vi "db filename.vi"(8 "error in (no error)":errorcluster, 10 "zDbName":string, 11 "db":dbl) -> (0 "error out":errorcluster, 2 "function return":string, 3 "db out":dbl)   [LabVIEW 2020, in "sqlite3.lvlib"]
uses:
  sqlite3.lvlib
  errstr.vi
  bin/sqlite3_64.dll
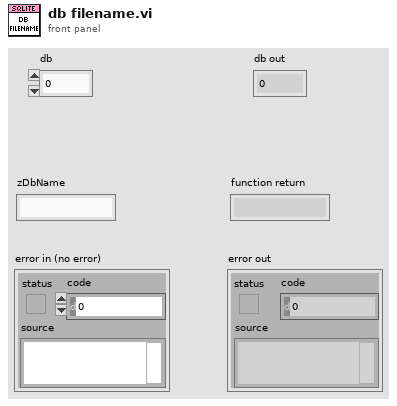
[diagram p1: front panel]
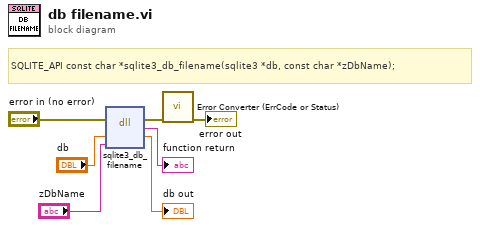
[diagram p0: block diagram]
diagram:
  # "SQLITE_API const char *sqlite3_db_filename(sqlite3 *db, const char *zDbName);"
  n1 = dll-call lib="C:/Users/Fred.Guo/Desktop/Database-configuration/externals/sqlite3/Source/bin/sqlite3_*.*" fn="sqlite3_db_filename"(error in="error in (no error)", "db"="db", "zDbName"="zDbName") -> (error out=w2:errorcluster, →"function return":string, "db"=→"db out":dbl)  [unwired: 3 in, 1 out]
  n2 = call "Error Converter (ErrCode or Status).vi"("error in (no error)"=w2) -> ("error out"=→"error out":errorcluster)  [unwired: 10 in]
